vi "find_preamble_new.vi"(0 "received \ntime symbol":cdb[][](array[numeric]), 5 "FFT Size":u32, 7 "CP Length":u32, 9 "1st preamble":cdb[](array[numeric]), 11 "2nd preamble":cdb[](array[numeric])) -> (4 "Received OFDM Symbol":cdb[](array[numeric]))   [LabVIEW 2014]
uses:
  <vilib>/Analysis/baseanly.llb/Complex A x B.vi
  <vilib>/Analysis/baseanly.llb/Complex A x Vector.vi
  <vilib>/Analysis/baseanly.llb/Complex Inverse Matrix.vi
  <vilib>/Analysis/NI_AALBase.lvlib
panel:
  out "output array":cdb[][](array[numeric])
  out "Array 2":i32[](array[numeric])
  out "x-y 2":i32
  out "max value 4":dbl
  out "max value 3":dbl
  out "Array":i32[](array[numeric])
  out "x-y":i32
  out "max value 2":dbl
  out "max value":dbl
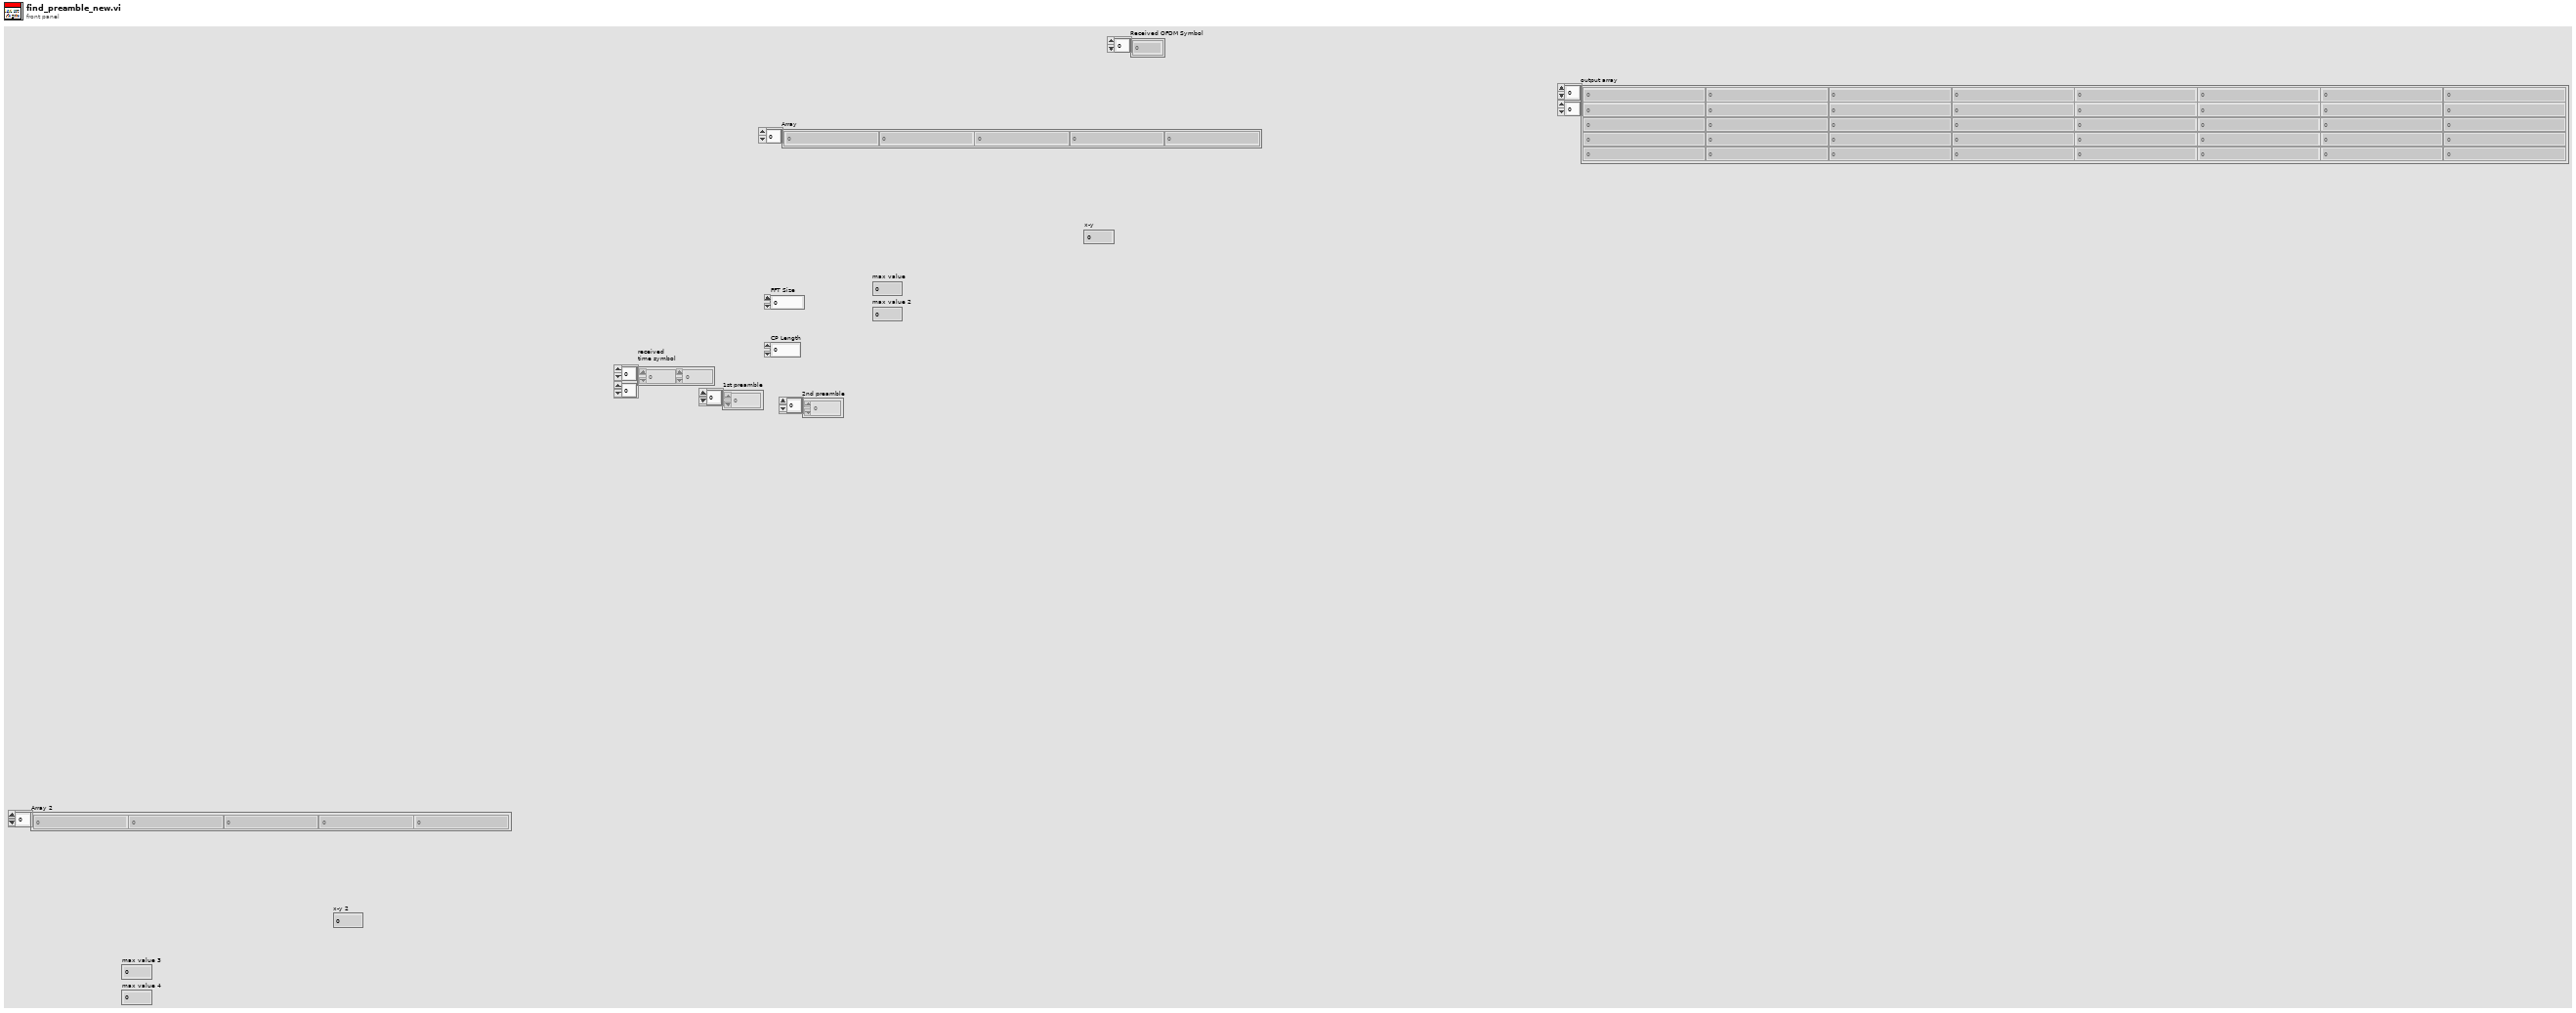
[diagram p1: front panel]
types:
  T1 = typedef "NI_Matrix.lvlib/ComplexMatrix.ctl" = cdb[][]
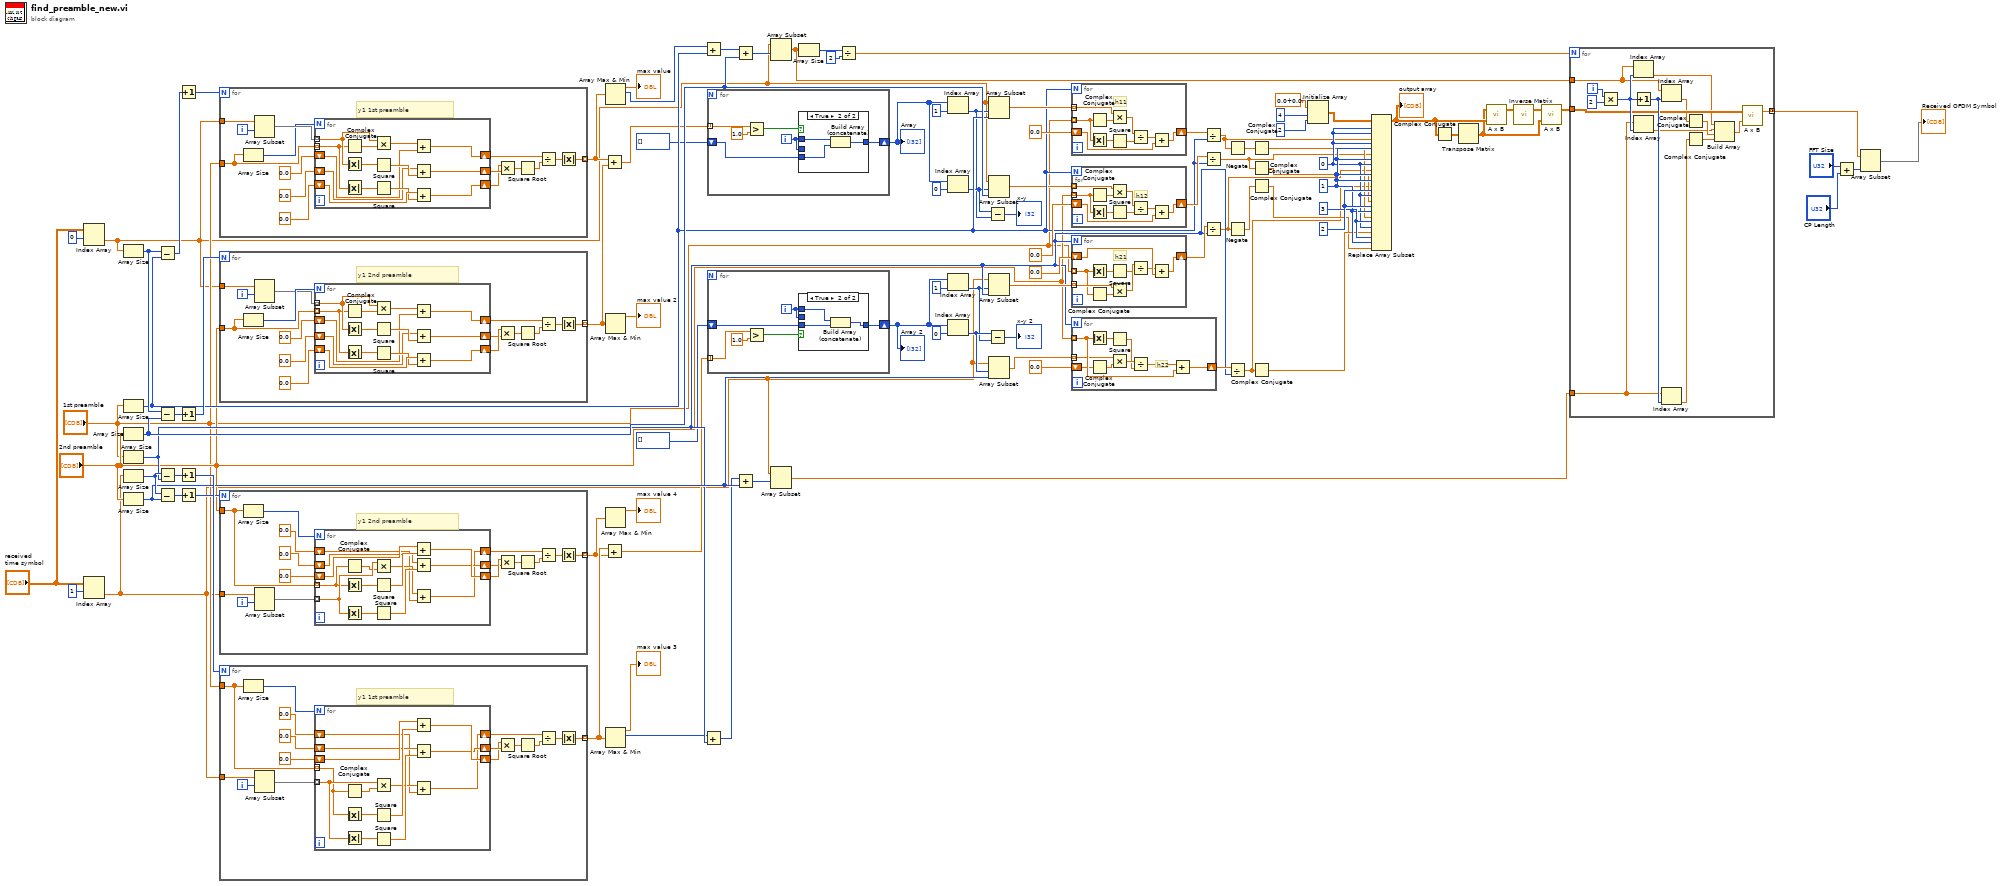
[diagram p0: block diagram]
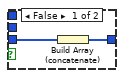
[diagram p2: hidden frame]
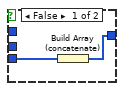
[diagram p3: hidden frame]
diagram:
  w25 = 3
  w26 = 2
  w24 = 1
  w23 = 0
  n1 = Index Array(array="received \ntime symbol", index (row)=0) -> (element=w32:cdb[])  [unwired: 1 in]
  n2 = Index Array(array="received \ntime symbol", index (row)=1) -> (element=w31:cdb[])  [unwired: 1 in]
  n3 = Array Size(array=w32) -> (size(s)=w93:i32)
  n4 = Array Size(array="1st preamble") -> (size(s)=w83:i32)
  n5 = Array Size(array="2nd preamble") -> (size(s)=w85:i32)
  n6 = Array Size(array="1st preamble") -> (size(s)=w53:i32)
  n7 = Array Size(array=w31) -> (size(s)=w61:i32)
  n8 = Array Size(array="2nd preamble") -> (size(s)=w55:i32)
  n9 = Subtract(x=w93, y=w83) -> (x-y=w97:i32)
  n10 = Subtract(x=w93, y=w85) -> (x-y=w95:i32)
  n11 = Subtract(x=w61, y=w53) -> (x-y=w65:i32)
  n12 = Subtract(x=w61, y=w55) -> (x-y=w63:i32)
  n13 = Increment(x=w97) -> (x+1=w96:i32)
  n14 = Increment(x=w95) -> (x+1=w94:i32)
  n15 = Increment(x=w65) -> (x+1=w64:i32)
  n16 = Increment(x=w63) -> (x+1=w62:i32)
  n17 = for {
    N: w96 -> [_]
    tunnel: w32 -> [w100]
    tunnel: "1st preamble" -> [w101]
    tunnel: [w99] -> w76 mode=indexing
    i -> [w98]
    # "y1 1st preamble"
    n18 = Array Size(array=w101) -> (size(s)=w102:i32)
    n19 = Array Subset(array=w100, index=w98) -> (w103:cdb[])  [unwired: 1 in]
    n20 = for {
      N: w102 -> [_]
      tunnel: w101 -> [w113] mode=indexing
      shift-right: [w123] -> w104
      shift-left: 0.0 -> [w125]
      shift-right: [w120] -> w105
      shift-left: 0.0 -> [w119]
      tunnel: w103 -> [w118] mode=indexing
      shift-right: [w114] -> w106
      shift-left: 0.0 -> [w115]
      n21 = Complex Conjugate(1:w113) -> (0:w117:cdb)
      n22 = Absolute Value(x=w118) -> (abs(x)=w122:dbl)
      n23 = Absolute Value(x=w113) -> (abs(x)=w126:dbl)
      n24 = Multiply(x=w118, y=w117) -> (x*y=w116:cdb)
      n25 = Square(x=w122) -> (x^2=w121:dbl)
      n26 = Square(x=w126) -> (x^2=w124:dbl)
      n27 = Add(x=w116, y=w115) -> (x+y=w114:cdb)
      n28 = Add(x=w119, y=w121) -> (x+y=w120:dbl)
      n29 = Add(x=w125, y=w124) -> (x+y=w123:dbl)
    }
    n30 = Multiply(x=w104, y=w105) -> (x*y=w108:dbl)
    n31 = Square Root(x=w108) -> (sqrt(x)=w109:dbl)
    n32 = Divide(x=w106, y=w109) -> (x/y=w107:cdb)
    n33 = Absolute Value(x=w107) -> (abs(x)=w99:dbl)
  }
  n34 = for {
    N: w94 -> [_]
    tunnel: "2nd preamble" -> [w127]
    tunnel: w32 -> [w128]
    tunnel: [w132] -> w75 mode=indexing
    i -> [w135]
    # "y1 2nd preamble"
    n35 = Array Size(array=w127) -> (size(s)=w141:i32)
    n36 = Array Subset(array=w128, index=w135) -> (w140:cdb[])  [unwired: 1 in]
    n37 = for {
      N: w141 -> [_]
      tunnel: w127 -> [w142] mode=indexing
      shift-right: [w152] -> w139
      shift-left: 0.0 -> [w154]
      shift-right: [w149] -> w138
      shift-left: 0.0 -> [w148]
      tunnel: w140 -> [w147] mode=indexing
      shift-right: [w143] -> w137
      shift-left: 0.0 -> [w144]
      n38 = Complex Conjugate(1:w142) -> (0:w146:cdb)
      n39 = Absolute Value(x=w147) -> (abs(x)=w151:dbl)
      n40 = Absolute Value(x=w142) -> (abs(x)=w155:dbl)
      n41 = Multiply(x=w147, y=w146) -> (x*y=w145:cdb)
      n42 = Square(x=w151) -> (x^2=w150:dbl)
      n43 = Square(x=w155) -> (x^2=w153:dbl)
      n44 = Add(x=w145, y=w144) -> (x+y=w143:cdb)
      n45 = Add(x=w148, y=w150) -> (x+y=w149:dbl)
      n46 = Add(x=w154, y=w153) -> (x+y=w152:dbl)
    }
    n47 = Multiply(x=w139, y=w138) -> (x*y=w134:dbl)
    n48 = Square Root(x=w134) -> (sqrt(x)=w133:dbl)
    n49 = Divide(x=w137, y=w133) -> (x/y=w136:cdb)
    n50 = Absolute Value(x=w136) -> (abs(x)=w132:dbl)
  }
  n51 = for {
    N: w62 -> [_]
    tunnel: "2nd preamble" -> [w156]
    tunnel: w31 -> [w157]
    tunnel: [w161] -> w45 mode=indexing
    i -> [w164]
    # "y1 2nd preamble"
    n52 = Array Size(array=w156) -> (size(s)=w170:i32)
    n53 = Array Subset(array=w157, index=w164) -> (w169:cdb[])  [unwired: 1 in]
    n54 = for {
      N: w170 -> [_]
      tunnel: w156 -> [w171] mode=indexing
      shift-right: [w181] -> w168
      shift-left: 0.0 -> [w183]
      shift-right: [w178] -> w167
      shift-left: 0.0 -> [w177]
      tunnel: w169 -> [w176] mode=indexing
      shift-right: [w172] -> w166
      shift-left: 0.0 -> [w173]
      n55 = Complex Conjugate(1:w171) -> (0:w175:cdb)
      n56 = Absolute Value(x=w171) -> (abs(x)=w184:dbl)
      n57 = Absolute Value(x=w176) -> (abs(x)=w180:dbl)
      n58 = Multiply(x=w176, y=w175) -> (x*y=w174:cdb)
      n59 = Square(x=w184) -> (x^2=w182:dbl)
      n60 = Square(x=w180) -> (x^2=w179:dbl)
      n61 = Add(x=w183, y=w182) -> (x+y=w181:dbl)
      n62 = Add(x=w177, y=w179) -> (x+y=w178:dbl)
      n63 = Add(x=w174, y=w173) -> (x+y=w172:cdb)
    }
    n64 = Multiply(x=w168, y=w167) -> (x*y=w163:dbl)
    n65 = Square Root(x=w163) -> (sqrt(x)=w162:dbl)
    n66 = Divide(x=w166, y=w162) -> (x/y=w165:cdb)
    n67 = Absolute Value(x=w165) -> (abs(x)=w161:dbl)
  }
  n68 = for {
    N: w64 -> [_]
    tunnel: w31 -> [w187]
    tunnel: "1st preamble" -> [w188]
    tunnel: [w186] -> w46 mode=indexing
    i -> [w185]
    # "y1 1st preamble"
    n69 = Array Size(array=w188) -> (size(s)=w189:i32)
    n70 = Array Subset(array=w187, index=w185) -> (w190:cdb[])  [unwired: 1 in]
    n71 = for {
      N: w189 -> [_]
      tunnel: w188 -> [w200] mode=indexing
      shift-right: [w210] -> w191
      shift-left: 0.0 -> [w212]
      shift-right: [w207] -> w192
      shift-left: 0.0 -> [w206]
      tunnel: w190 -> [w205] mode=indexing
      shift-right: [w201] -> w193
      shift-left: 0.0 -> [w202]
      n72 = Complex Conjugate(1:w200) -> (0:w204:cdb)
      n73 = Absolute Value(x=w200) -> (abs(x)=w213:dbl)
      n74 = Absolute Value(x=w205) -> (abs(x)=w209:dbl)
      n75 = Multiply(x=w205, y=w204) -> (x*y=w203:cdb)
      n76 = Square(x=w213) -> (x^2=w211:dbl)
      n77 = Square(x=w209) -> (x^2=w208:dbl)
      n78 = Add(x=w212, y=w211) -> (x+y=w210:dbl)
      n79 = Add(x=w206, y=w208) -> (x+y=w207:dbl)
      n80 = Add(x=w203, y=w202) -> (x+y=w201:cdb)
    }
    n81 = Multiply(x=w191, y=w192) -> (x*y=w195:dbl)
    n82 = Square Root(x=w195) -> (sqrt(x)=w196:dbl)
    n83 = Divide(x=w193, y=w196) -> (x/y=w194:cdb)
    n84 = Absolute Value(x=w194) -> (abs(x)=w186:dbl)
  }
  n85 = Add(x=w76, y=w75) -> (x+y=w74:dbl[])
  n86 = Add(x=w46, y=w45) -> (x+y=w44:dbl[])
  n87 = Array Max & Min(array=w76) -> (max value=→"max value":dbl, max index (indices)=w77:i32)  [unwired: 2 out]
  n88 = Array Max & Min(array=w75) -> (max value=→"max value 2":dbl)  [unwired: 3 out]
  n89 = Array Max & Min(array=w45) -> (max value=→"max value 4":dbl)  [unwired: 3 out]
  n90 = Array Max & Min(array=w46) -> (max value=→"max value 3":dbl, max index (indices)=w47:i32)  [unwired: 2 out]
  n91 = Add(x=w77, y=w83) -> (x+y=w84:i32)
  n92 = Add(x=w47, y=w53) -> (x+y=w54:i32)
  n93 = for {
    tunnel: w74 -> [w219] mode=indexing
    shift-right: [w216] -> w71
    shift-left: i32[] [] -> [w215]
    i -> [w214]
    n94 = Greater?(x=w219, y=1.0) -> (0:w217:bool)
    n95 = case shown="True" w217 {
      tunnel: w214 -> [_ _]
      tunnel: [w221 w224] -> w216
      tunnel: w215 -> [w220 w222]
      tunnel: w214 -> [_ w223]
      frame False {
        n96 = Build Array (concatenate)(w220) -> (w221:i32[])
      }
      frame True {
        n97 = Build Array (concatenate)(w223, w222) -> (w224:i32[])
      }
    }
  }
  "Array" <- w71
  n98 = for {
    tunnel: w44 -> [w230] mode=indexing
    shift-right: [w227] -> w41
    shift-left: i32[] [] -> [w226]
    i -> [w225]
    n99 = Greater?(x=w230, y=1.0) -> (0:w228:bool)
    n100 = case shown="True" w228 {
      tunnel: w225 -> [_ _]
      tunnel: [w232 w235] -> w227
      tunnel: w226 -> [w231 w233]
      tunnel: w225 -> [_ w234]
      frame False {
        n101 = Build Array (concatenate)(w231) -> (w232:i32[])
      }
      frame True {
        n102 = Build Array (concatenate)(w234, w233) -> (w235:i32[])
      }
    }
  }
  "Array 2" <- w41
  n103 = Add(x=w84, y=w85) -> (x+y=w82:i32)
  n104 = Add(x=w54, y=w55) -> (x+y=w52:i32)
  n105 = Array Subset(array=w32, index=w82) -> (w5:cdb[])  [unwired: 1 in]
  n106 = Array Subset(array=w31, index=w52) -> (w4:cdb[])  [unwired: 1 in]
  n107 = Array Size(array=w5) -> (size(s)=w92:i32)
  n108 = Divide(x=w92, y=2) -> (x/y=w3:dbl)
  n109 = Index Array(array=w71, index=1) -> (element=w68:i32)
  n110 = Index Array(array=w71, index=0) -> (element=w69:i32)
  n111 = Index Array(array=w41, index=1) -> (element=w38:i32)
  n112 = Index Array(array=w41, index=0) -> (element=w39:i32)
  n113 = Subtract(x=w69, y=w68) -> (x-y=→"x-y":i32)
  n114 = Subtract(x=w39, y=w38) -> (x-y=→"x-y 2":i32)
  n115 = Array Subset(array=w32, index=w68, length=w83) -> (w86:cdb[])
  n116 = Array Subset(array=w32, index=w69, length=w85) -> (w81:cdb[])
  n117 = Array Subset(array=w31, index=w38, length=w53) -> (w56:cdb[])
  n118 = Array Subset(array=w31, index=w39, length=w55) -> (w51:cdb[])
  n119 = for {
    N: w83 -> [_]
    shift-right: [w237] -> w90
    shift-left: 0.0 -> [w239]
    tunnel: w86 -> [w242] mode=indexing
    tunnel: "1st preamble" -> [w236] mode=indexing
    # "h11"
    n120 = Complex Conjugate(1:w236) -> (0:w244:cdb)
    n121 = Absolute Value(x=w236) -> (abs(x)=w243:dbl)
    n122 = Square(x=w243) -> (x^2=w240:dbl)
    n123 = Multiply(x=w242, y=w244) -> (x*y=w241:cdb)
    n124 = Divide(x=w241, y=w240) -> (x/y=w238:cdb)
    n125 = Add(x=w238, y=w239) -> (x+y=w237:cdb)
  }
  n126 = for {
    N: w83 -> [_]
    shift-right: [w247] -> w88
    shift-left: 0.0 -> [w249]
    tunnel: "2nd preamble" -> [w246] mode=indexing
    tunnel: w81 -> [w245] mode=indexing
    # "h12"
    n127 = Complex Conjugate(1:w246) -> (0:w253:cdb)
    n128 = Absolute Value(x=w246) -> (abs(x)=w252:dbl)
    n129 = Square(x=w252) -> (x^2=w250:dbl)
    n130 = Multiply(x=w245, y=w253) -> (x*y=w251:cdb)
    n131 = Divide(x=w251, y=w250) -> (x/y=w248:cdb)
    n132 = Add(x=w248, y=w249) -> (x+y=w247:cdb)
  }
  n133 = for {
    N: w53 -> [_]
    shift-right: [w255] -> w60
    shift-left: 0.0 -> [w257]
    tunnel: w56 -> [w260] mode=indexing
    tunnel: "1st preamble" -> [w254] mode=indexing
    # "h21"
    n134 = Absolute Value(x=w254) -> (abs(x)=w261:dbl)
    n135 = Complex Conjugate(1:w254) -> (0:w262:cdb)
    n136 = Square(x=w261) -> (x^2=w258:dbl)
    n137 = Multiply(x=w260, y=w262) -> (x*y=w259:cdb)
    n138 = Divide(x=w259, y=w258) -> (x/y=w256:cdb)
    n139 = Add(x=w256, y=w257) -> (x+y=w255:cdb)
  }
  n140 = for {
    N: w53 -> [_]
    shift-right: [w265] -> w58
    shift-left: 0.0 -> [w267]
    tunnel: "2nd preamble" -> [w264] mode=indexing
    tunnel: w51 -> [w263] mode=indexing
    # "h22"
    n141 = Absolute Value(x=w264) -> (abs(x)=w270:dbl)
    n142 = Complex Conjugate(1:w264) -> (0:w271:cdb)
    n143 = Square(x=w270) -> (x^2=w268:dbl)
    n144 = Multiply(x=w263, y=w271) -> (x*y=w269:cdb)
    n145 = Divide(x=w269, y=w268) -> (x/y=w266:cdb)
    n146 = Add(x=w266, y=w267) -> (x+y=w265:cdb)
  }
  n147 = Divide(x=w90, y=w83) -> (x/y=w8:cdb)
  n148 = Divide(x=w88, y=w83) -> (x/y=w9:cdb)
  n149 = Divide(x=w60, y=w53) -> (x/y=w6:cdb)
  n150 = Negate(x=w8) -> (-x=w11:cdb)
  n151 = Negate(x=w6) -> (-x=w10:cdb)
  n152 = Divide(x=w58, y=w53) -> (x/y=w7:cdb)
  n153 = Complex Conjugate(1:w11) -> (0:w14:cdb)
  n154 = Complex Conjugate(1:w9) -> (0:w15:cdb)
  n155 = Complex Conjugate(1:w10) -> (0:w12:cdb)
  n156 = Complex Conjugate(1:w7) -> (0:w13:cdb)
  n157 = Initialize Array(cdb 0.0+0.0i, 4, 2) -> (w27:cdb[][])
  n158 = Replace Array Subset(array=w27, new element #1=w8, index (row) #1=w23, index (col) #1=w23, new element #2=w9, index (row) #2=w23, index (col) #2=w24, new element #3=w6, index (row) #3=w24, index (col) #3=w23, new element #4=w7, index (row) #4=w24, index (col) #4=w24, new element #5=w15, index (row) #5=w26, index (col) #5=w23, new element #6=w14, index (row) #6=w26, index (col) #6=w24, new element #7=w13, index (row) #7=w25, index (col) #7=w23, new element #8=w12, index (row) #8=w25, index (col) #8=w24) -> (w20:cdb[][])
  "output array" <- w20
  n159 = Complex Conjugate(1:w20) -> (0:w21:cdb[][])
  n160 = Transpose Matrix(1:w21) -> (0:w18:cdb[][])
  n161 = call-poly <vilib>:"A x B.vi"("B"=w20, "A"=w18) -> ("A x B"=w19:T1)  [unwired: 1 out]
  n162 = call-poly <vilib>:"Inverse Matrix.vi"("Input Matrix"=w19) -> ("Inverse Matrix"=w16:T1)  [unwired: 1 in, 1 out]
  n163 = call-poly <vilib>:"A x B.vi"("B"=w18, "A"=w16) -> ("A x B"=w17:T1)  [unwired: 1 out]
  n164 = for {
    N: w3 -> [_]
    tunnel: w17 -> [w280]
    tunnel: [w278] -> w2 mode=concatenating
    tunnel: w5 -> [w277]
    tunnel: w4 -> [w276]
    i -> [w286]
    n165 = Multiply(x=w286, y=2) -> (x*y=w284:i32)
    n166 = Index Array(array=w277, index=w284) -> (element=w275:cdb)
    n167 = Increment(x=w284) -> (x+1=w283:i32)
    n168 = Index Array(array=w276, index=w284) -> (element=w274:cdb)
    n169 = Index Array(array=w277, index=w283) -> (element=w273:cdb)
    n170 = Index Array(array=w276, index=w283) -> (element=w272:cdb)
    n171 = Complex Conjugate(1:w273) -> (0:w282:cdb)
    n172 = Complex Conjugate(1:w272) -> (0:w281:cdb)
    n173 = Build Array(w275, w274, w282, w281) -> (w279:cdb[])
    n174 = call-poly <vilib>:"A x B.vi"("Vector"=w279, "A"=w280) -> ("A x Vector"=w278:cdb[])  [unwired: 1 out]
  }
  n175 = Add(x="FFT Size", y="CP Length") -> (x+y=w30:u32)
  n176 = Array Subset(array=w2, length=w30) -> (→"Received OFDM Symbol":cdb[])  [unwired: 1 in]
